vi "All IOs 2.vi"() -> ()   [LabVIEW 2012]
uses:
  <vilib>/eio/EIONode/EIONode.xnode
  <vilib>/rvi/eio/common/nirviEmuTemplateMethod_errors.vi
panel:
  in  "6DOF robot arm controls":T1={"Axis  1 (base)"=500, "Axis 2"=500, "Axis 3"=500, "Axis 4"=500, "Axis 5"=500, "Axis 6 (claw)"=500} {"Axis 6 (claw)" min=500 max=2000; "Axis 5" min=500 max=2000; "Axis 4" min=500 max=2000; "Axis 3" min=500 max=2000; "Axis 2" min=500 max=2000; "Axis  1 (base)" min=500 max=2000}
  out "Time of flight":T2
  in  "LF":bool
  in  "LB":bool
  in  "RF":bool
  in  "RB":bool
  in  "ESC Pulse Duration (uS)":u16=1000 min=1000 max=2000
  in  "Servo Angle (500-2000)":u16=1000 min=500 max=2000
  out "Lipo Battery Voltage":i16
  out "PIR 2":bool
  in  "On-board LED Brightness":T3 {"LED3 Brightness" max=100; "LED2 Brightness" max=100; "LED1 Brightness" max=100; "LED0 Brightness" max=100}
  out "Accelerometer":T4
  out "Button0":bool
  out "PIR":bool
  out "IR Sensors":T5
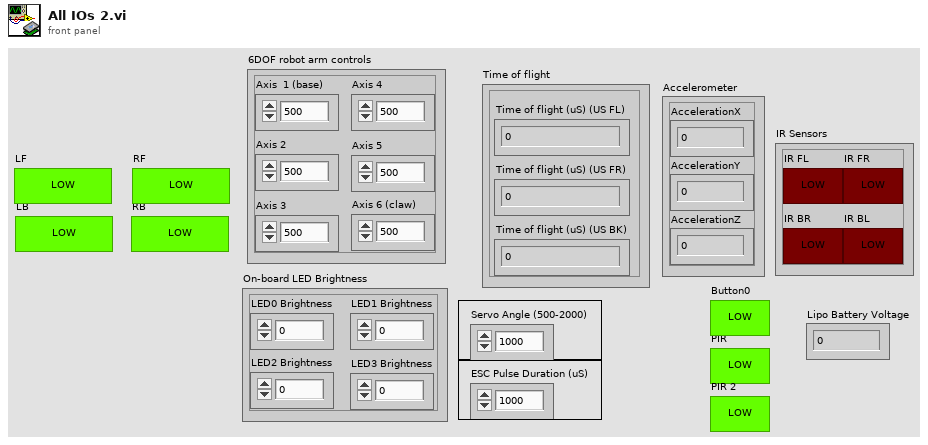
[diagram p1: front panel]
types:
  T1 = cluster{"Axis  1 (base)":i16, "Axis 2":i16, "Axis 3":i16, "Axis 4":i16, "Axis 5":i16, "Axis 6 (claw)":i16}
  T2 = cluster{"Time of flight (uS) (US FL)":u32, "Time of flight (uS) (US FR)":u32, "Time of flight (uS) (US BK)":u32}
  T3 = cluster{"LED0 Brightness":u8, "LED1 Brightness":u8, "LED2 Brightness":u8, "LED3 Brightness":u8}
  T4 = cluster{"AccelerationX":i16, "AccelerationY":i16, "AccelerationZ":i16}
  T5 = cluster{"IR FL":bool, "IR FR":bool, "IR BR":bool, "IR BL":bool}
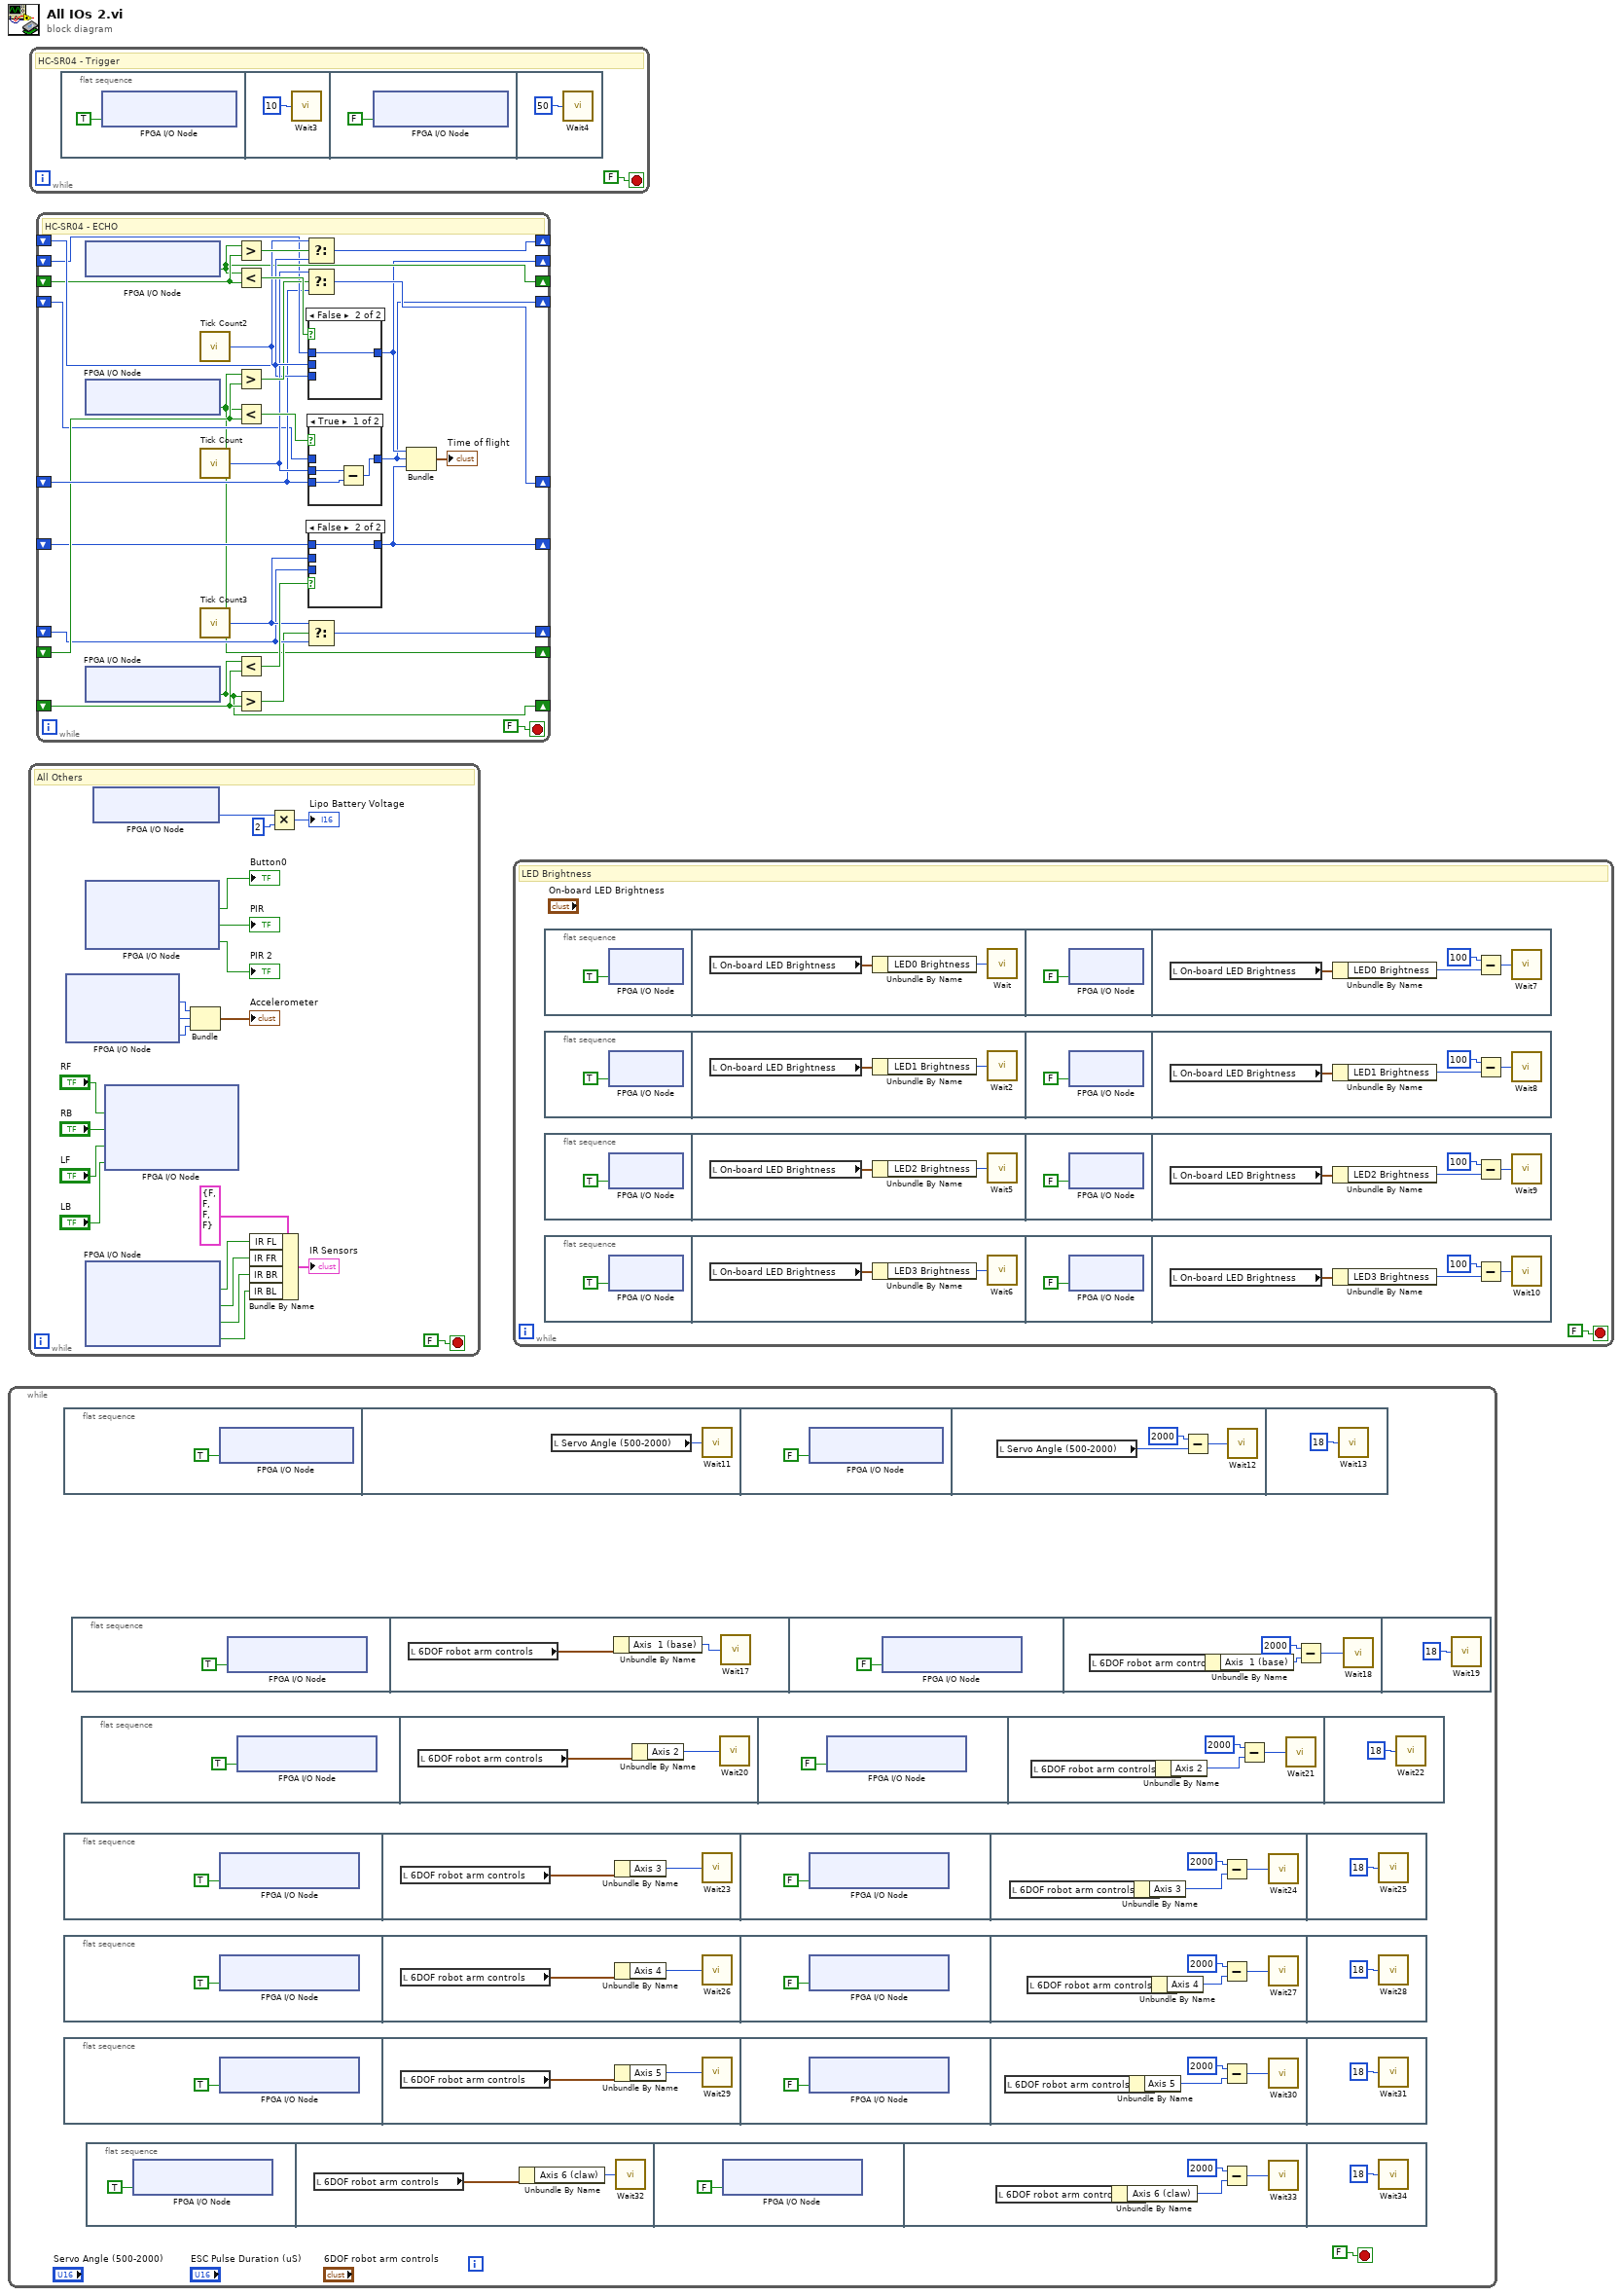
[diagram p0: block diagram]
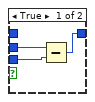
[diagram p2: hidden frame]
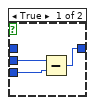
[diagram p3: hidden frame]
diagram:
  n1 = while {
    stop <- FALSE stop-if-true
    n2 = flat-sequence {
      frame #0 {
        n3 = xnode "FPGA I/O Node"("ConnectorB/DIO8"=TRUE) -> ()  [unwired: 1 in, 1 out]
      }
      frame #1 {
        n4 = local read "Servo Angle (500-2000)"() -> (w57:u16)
        n5 = call "Wait11"("Count(uSec)"=w57) -> ()  [unwired: 1 out]
      }
      frame #2 {
        n6 = xnode "FPGA I/O Node"("ConnectorB/DIO8"=FALSE) -> ()  [unwired: 1 in, 1 out]
      }
      frame #3 {
        n7 = local read "Servo Angle (500-2000)"() -> (w60:u16)
        n8 = Subtract(x=i16 2000, y=w60) -> (x-y=w59:u16)
        n9 = call "Wait12"("Count(uSec)"=w59) -> ()  [unwired: 1 out]
      }
      frame #4 {
        n10 = call "Wait13"("Count(mSec)"=u32 18) -> ()  [unwired: 1 out]
      }
    }
    n11 = flat-sequence {
      frame #0 {
        n12 = xnode "FPGA I/O Node"("ConnectorB/DIO12"=TRUE) -> ()  [unwired: 1 in, 1 out]
      }
      frame #1 {
        n13 = local read "6DOF robot arm controls"() -> (w31:T1)
        n14 = Unbundle By Name(w31) -> ("Axis 3"=w30:i16)
        n15 = call "Wait23"("Count(uSec)"=w30) -> ()  [unwired: 1 out]
      }
      frame #2 {
        n16 = xnode "FPGA I/O Node"("ConnectorB/DIO12"=FALSE) -> ()  [unwired: 1 in, 1 out]
      }
      frame #3 {
        n17 = local read "6DOF robot arm controls"() -> (w34:T1)
        n18 = Unbundle By Name(w34) -> ("Axis 3"=w33:i16)
        n19 = Subtract(x=i16 2000, y=w33) -> (x-y=w35:i16)
        n20 = call "Wait24"("Count(uSec)"=w35) -> ()  [unwired: 1 out]
      }
      frame #4 {
        n21 = call "Wait25"("Count(mSec)"=u32 18) -> ()  [unwired: 1 out]
      }
    }
    n22 = flat-sequence {
      frame #0 {
        n23 = xnode "FPGA I/O Node"("ConnectorB/DIO13"=TRUE) -> ()  [unwired: 1 in, 1 out]
      }
      frame #1 {
        n24 = local read "6DOF robot arm controls"() -> (w22:T1)
        n25 = Unbundle By Name(w22) -> ("Axis 4"=w21:i16)
        n26 = call "Wait26"("Count(uSec)"=w21) -> ()  [unwired: 1 out]
      }
      frame #2 {
        n27 = xnode "FPGA I/O Node"("ConnectorB/DIO13"=FALSE) -> ()  [unwired: 1 in, 1 out]
      }
      frame #3 {
        n28 = local read "6DOF robot arm controls"() -> (w25:T1)
        n29 = Unbundle By Name(w25) -> ("Axis 4"=w24:i16)
        n30 = Subtract(x=i16 2000, y=w24) -> (x-y=w26:i16)
        n31 = call "Wait27"("Count(uSec)"=w26) -> ()  [unwired: 1 out]
      }
      frame #4 {
        n32 = call "Wait28"("Count(mSec)"=u32 18) -> ()  [unwired: 1 out]
      }
    }
    n33 = flat-sequence {
      frame #0 {
        n34 = xnode "FPGA I/O Node"("ConnectorB/DIO14"=TRUE) -> ()  [unwired: 1 in, 1 out]
      }
      frame #1 {
        n35 = local read "6DOF robot arm controls"() -> (w13:T1)
        n36 = Unbundle By Name(w13) -> ("Axis 5"=w12:i16)
        n37 = call "Wait29"("Count(uSec)"=w12) -> ()  [unwired: 1 out]
      }
      frame #2 {
        n38 = xnode "FPGA I/O Node"("ConnectorB/DIO14"=FALSE) -> ()  [unwired: 1 in, 1 out]
      }
      frame #3 {
        n39 = local read "6DOF robot arm controls"() -> (w16:T1)
        n40 = Unbundle By Name(w16) -> ("Axis 5"=w15:i16)
        n41 = Subtract(x=i16 2000, y=w15) -> (x-y=w17:i16)
        n42 = call "Wait30"("Count(uSec)"=w17) -> ()  [unwired: 1 out]
      }
      frame #4 {
        n43 = call "Wait31"("Count(mSec)"=u32 18) -> ()  [unwired: 1 out]
      }
    }
    n44 = flat-sequence {
      frame #0 {
        n45 = xnode "FPGA I/O Node"("ConnectorB/DIO10"=TRUE) -> ()  [unwired: 1 in, 1 out]
      }
      frame #1 {
        n46 = local read "6DOF robot arm controls"() -> (w49:T1)
        n47 = Unbundle By Name(w49) -> ("Axis  1 (base)"=w48:i16)
        n48 = call "Wait17"("Count(uSec)"=w48) -> ()  [unwired: 1 out]
      }
      frame #2 {
        n49 = xnode "FPGA I/O Node"("ConnectorB/DIO10"=FALSE) -> ()  [unwired: 1 in, 1 out]
      }
      frame #3 {
        n50 = local read "6DOF robot arm controls"() -> (w52:T1)
        n51 = Unbundle By Name(w52) -> ("Axis  1 (base)"=w51:i16)
        n52 = Subtract(x=i16 2000, y=w51) -> (x-y=w53:i16)
        n53 = call "Wait18"("Count(uSec)"=w53) -> ()  [unwired: 1 out]
      }
      frame #4 {
        n54 = call "Wait19"("Count(mSec)"=u32 18) -> ()  [unwired: 1 out]
      }
    }
    n55 = flat-sequence {
      frame #0 {
        n56 = xnode "FPGA I/O Node"("ConnectorB/DIO11"=TRUE) -> ()  [unwired: 1 in, 1 out]
      }
      frame #1 {
        n57 = local read "6DOF robot arm controls"() -> (w40:T1)
        n58 = Unbundle By Name(w40) -> ("Axis 2"=w39:i16)
        n59 = call "Wait20"("Count(uSec)"=w39) -> ()  [unwired: 1 out]
      }
      frame #2 {
        n60 = xnode "FPGA I/O Node"("ConnectorB/DIO11"=FALSE) -> ()  [unwired: 1 in, 1 out]
      }
      frame #3 {
        n61 = local read "6DOF robot arm controls"() -> (w43:T1)
        n62 = Unbundle By Name(w43) -> ("Axis 2"=w42:i16)
        n63 = Subtract(x=i16 2000, y=w42) -> (x-y=w44:i16)
        n64 = call "Wait21"("Count(uSec)"=w44) -> ()  [unwired: 1 out]
      }
      frame #4 {
        n65 = call "Wait22"("Count(mSec)"=u32 18) -> ()  [unwired: 1 out]
      }
    }
    n66 = flat-sequence {
      frame #0 {
        n67 = xnode "FPGA I/O Node"("ConnectorB/DIO15"=TRUE) -> ()  [unwired: 1 in, 1 out]
      }
      frame #1 {
        n68 = local read "6DOF robot arm controls"() -> (w4:T1)
        n69 = Unbundle By Name(w4) -> ("Axis 6 (claw)"=w3:i16)
        n70 = call "Wait32"("Count(uSec)"=w3) -> ()  [unwired: 1 out]
      }
      frame #2 {
        n71 = xnode "FPGA I/O Node"("ConnectorB/DIO15"=FALSE) -> ()  [unwired: 1 in, 1 out]
      }
      frame #3 {
        n72 = local read "6DOF robot arm controls"() -> (w7:T1)
        n73 = Unbundle By Name(w7) -> ("Axis 6 (claw)"=w6:i16)
        n74 = Subtract(x=i16 2000, y=w6) -> (x-y=w8:i16)
        n75 = call "Wait33"("Count(uSec)"=w8) -> ()  [unwired: 1 out]
      }
      frame #4 {
        n76 = call "Wait34"("Count(mSec)"=u32 18) -> ()  [unwired: 1 out]
      }
    }
  }
  n77 = while {
    stop <- FALSE stop-if-true
    # "All Others"
    n78 = xnode "FPGA I/O Node"() -> ("AccelerationX"=w83:i16, "AccelerationY"=w82:i16, "AccelerationZ"=w81:i16)  [unwired: 3 in, 3 out]
    n79 = xnode "FPGA I/O Node"() -> ("Button0"=→"Button0":bool, "ConnectorB/DIO4"=→"PIR":bool, "ConnectorB/DIO5"=→"PIR 2":bool)  [unwired: 3 in, 3 out]
    n80 = xnode "FPGA I/O Node"() -> ("ConnectorC/DIO4"=w74:bool, "ConnectorC/DIO5"=w73:bool, "ConnectorC/DIO6"=w72:bool, "ConnectorC/DIO7"=w71:bool)  [unwired: 4 in, 4 out]
    n81 = xnode "FPGA I/O Node"() -> ("ConnectorC/AI0"=w69:i16)  [unwired: 1 in, 1 out]
    n82 = xnode "FPGA I/O Node"("ConnectorB/DIO0"="RF", "ConnectorB/DIO1"="RB", "ConnectorB/DIO2"="LF", "ConnectorB/DIO3"="LB") -> ()  [unwired: 4 in, 4 out]
    n83 = Bundle("AccelerationX"=w83, "AccelerationY"=w82, "AccelerationZ"=w81) -> (→"Accelerometer":T4)  [unwired: 1 in]
    n84 = Bundle By Name(cluster=T5 {"IR FL"=FALSE, "IR FR"=FALSE, "IR BR"=FALSE, "IR BL"=FALSE} ("IR Sensors 2"), "IR FL"=w74, "IR FR"=w73, "IR BR"=w72, "IR BL"=w71) -> (→"IR Sensors":T5)
    n85 = Multiply(x=w69, y=i16 2) -> (x*y=→"Lipo Battery Voltage":i16)
  }
  n86 = while {
    stop <- FALSE stop-if-true
    # "HC-SR04 - Trigger"
    n87 = flat-sequence {
      frame #0 {
        n88 = xnode "FPGA I/O Node"("ConnectorC/DIO0"=TRUE ("ConnectorC/DIO6")) -> ()  [unwired: 1 in, 1 out]
      }
      frame #1 {
        n89 = call "Wait3"("Count(uSec)"=u32 10) -> ()  [unwired: 1 out]
      }
      frame #2 {
        n90 = xnode "FPGA I/O Node"("ConnectorC/DIO0"=FALSE ("ConnectorC/DIO6")) -> ()  [unwired: 1 in, 1 out]
      }
      frame #3 {
        n91 = call "Wait4"("Count(mSec)"=i16 50) -> ()  [unwired: 1 out]
      }
    }
  }
  n92 = while {
    shift-right: [w109] -> _
    shift-left: _ -> [w110]
    shift-right: [w107] -> _
    shift-left: _ -> [w108]
    shift-right: [w92] -> _
    shift-left: _ -> [w106]
    shift-right: [w102] -> _
    shift-left: _ -> [w105]
    shift-right: [w95] -> _
    shift-left: _ -> [w104]
    shift-right: [w91] -> _
    shift-left: _ -> [w103]
    shift-right: [w90] -> _
    shift-left: _ -> [w101]
    shift-right: [w98] -> _
    shift-left: _ -> [w99]
    shift-right: [w94] -> _
    shift-left: _ -> [w97]
    stop <- FALSE stop-if-true
    # "HC-SR04 - ECHO"
    n93 = xnode "FPGA I/O Node"() -> ("ConnectorC/DIO1"=w107:bool)  [unwired: 1 in, 1 out]
    n94 = xnode "FPGA I/O Node"() -> ("ConnectorC/DIO2"=w95:bool)  [unwired: 1 in, 1 out]
    n95 = xnode "FPGA I/O Node"() -> ("ConnectorC/DIO3"=w94:bool)  [unwired: 1 in, 1 out]
    n96 = call "Tick Count2"() -> ("Tick Count(uSec)"=w114:u32)
    n97 = call "Tick Count"() -> ("Tick Count(uSec)"=w111:u32)
    n98 = call "Tick Count3"() -> ("Tick Count(uSec)"=w100:u32)
    n99 = Greater?(x=w107, y=w108) -> (0:w116:bool)
    n100 = Less?(x=w107, y=w108) -> (x < y?=w115:bool)
    n101 = Greater?(x=w95, y=w104) -> (0:w113:bool)
    n102 = Less?(x=w95, y=w104) -> (x < y?=w112:bool)
    n103 = Less?(x=w94, y=w97) -> (x < y?=w117:bool)
    n104 = Greater?(x=w94, y=w97) -> (0:w96:bool)
    n105 = Select(t=w114, s=w116, f=w110) -> (s? t:f=w109:u32)
    n106 = Select(t=w111, s=w113, f=w105) -> (s? t:f=w102:u32)
    n107 = Select(t=w100, s=w96, f=w99) -> (s? t:f=w98:u32)
    n108 = case shown="False" w115 {
      tunnel: w106 -> [_ w125]
      tunnel: w114 -> [w122 _]
      tunnel: w110 -> [w123 _]
      tunnel: [w124 w125] -> w92
      frame True {
        n109 = Subtract(x=w122, y=w123) -> (x-y=w124:u32)
      }
      frame False {
      }
    }
    n110 = case shown="True" w112 {
      tunnel: w103 -> [_ w129]
      tunnel: w111 -> [w126 _]
      tunnel: w105 -> [w127 _]
      tunnel: [w128 w129] -> w91
      frame True {
        n111 = Subtract(x=w126, y=w127) -> (x-y=w128:u32)
      }
      frame False {
      }
    }
    n112 = case shown="False" w117 {
      tunnel: w101 -> [_ w121]
      tunnel: w100 -> [w118 _]
      tunnel: w99 -> [w119 _]
      tunnel: [w120 w121] -> w90
      frame True {
        n113 = Subtract(x=w118, y=w119) -> (x-y=w120:u32)
      }
      frame False {
      }
    }
    n114 = Bundle(w92, w91, w90) -> (→"Time of flight":cluster{u32, u32, u32})  [unwired: 1 in]
  }
  n115 = while {
    stop <- FALSE stop-if-true
    # "LED Brightness"
    n116 = flat-sequence {
      frame #0 {
        n117 = xnode "FPGA I/O Node"("LED0"=TRUE) -> ()  [unwired: 1 in, 1 out]
      }
      frame #1 {
        n118 = local read "On-board LED Brightness"() -> (w157:T3)
        n119 = Unbundle By Name(w157) -> ("LED0 Brightness"=w156:u8)
        n120 = call "Wait"("Count(uSec)"=w156) -> ()  [unwired: 1 out]
      }
      frame #2 {
        n121 = xnode "FPGA I/O Node"("LED0"=FALSE) -> ()  [unwired: 1 in, 1 out]
      }
      frame #3 {
        n122 = local read "On-board LED Brightness"() -> (w162:T3)
        n123 = Unbundle By Name(w162) -> ("LED0 Brightness"=w159:u8)
        n124 = Subtract(x=i16 100, y=w159) -> (x-y=w161:i16)
        n125 = call "Wait7"("Count(uSec)"=w161) -> ()  [unwired: 1 out]
      }
    }
    n126 = flat-sequence {
      frame #0 {
        n127 = xnode "FPGA I/O Node"("LED1"=TRUE) -> ()  [unwired: 1 in, 1 out]
      }
      frame #1 {
        n128 = local read "On-board LED Brightness"() -> (w148:T3)
        n129 = Unbundle By Name(w148) -> ("LED1 Brightness"=w149:u8)
        n130 = call "Wait2"("Count(uSec)"=w149) -> ()  [unwired: 1 out]
      }
      frame #2 {
        n131 = xnode "FPGA I/O Node"("LED1"=FALSE) -> ()  [unwired: 1 in, 1 out]
      }
      frame #3 {
        n132 = local read "On-board LED Brightness"() -> (w154:T3)
        n133 = Unbundle By Name(w154) -> ("LED1 Brightness"=w153:u8)
        n134 = Subtract(x=i16 100, y=w153) -> (x-y=w152:i16)
        n135 = call "Wait8"("Count(uSec)"=w152) -> ()  [unwired: 1 out]
      }
    }
    n136 = flat-sequence {
      frame #0 {
        n137 = xnode "FPGA I/O Node"("LED2"=TRUE) -> ()  [unwired: 1 in, 1 out]
      }
      frame #1 {
        n138 = local read "On-board LED Brightness"() -> (w141:T3)
        n139 = Unbundle By Name(w141) -> ("LED2 Brightness"=w140:u8)
        n140 = call "Wait5"("Count(uSec)"=w140) -> ()  [unwired: 1 out]
      }
      frame #2 {
        n141 = xnode "FPGA I/O Node"("LED2"=FALSE) -> ()  [unwired: 1 in, 1 out]
      }
      frame #3 {
        n142 = local read "On-board LED Brightness"() -> (w146:T3)
        n143 = Unbundle By Name(w146) -> ("LED2 Brightness"=w143:u8)
        n144 = Subtract(x=i16 100, y=w143) -> (x-y=w145:i16)
        n145 = call "Wait9"("Count(uSec)"=w145) -> ()  [unwired: 1 out]
      }
    }
    n146 = flat-sequence {
      frame #0 {
        n147 = xnode "FPGA I/O Node"("LED3"=TRUE) -> ()  [unwired: 1 in, 1 out]
      }
      frame #1 {
        n148 = local read "On-board LED Brightness"() -> (w132:T3)
        n149 = Unbundle By Name(w132) -> ("LED3 Brightness"=w133:u8)
        n150 = call "Wait6"("Count(uSec)"=w133) -> ()  [unwired: 1 out]
      }
      frame #2 {
        n151 = xnode "FPGA I/O Node"("LED3"=FALSE) -> ()  [unwired: 1 in, 1 out]
      }
      frame #3 {
        n152 = local read "On-board LED Brightness"() -> (w138:T3)
        n153 = Unbundle By Name(w138) -> ("LED3 Brightness"=w135:u8)
        n154 = Subtract(x=i16 100, y=w135) -> (x-y=w137:i16)
        n155 = call "Wait10"("Count(uSec)"=w137) -> ()  [unwired: 1 out]
      }
    }
  }
